vi "Copy Builds To NIVS Dir.vi"(5 "Files Generated by Build":path[](array[path]), 6 "Top Level/Always Included VIs":path[](array[path]), 7 "Destination Path":path, 8 "error in (no error)":errorcluster, 9 "Target Name":string, 10 "Build Specification Name":string, 11 "Project Path":path) -> (0 "error out":errorcluster)   [LabVIEW 2020]
uses:
  <vilib>/Utility/sysdir.llb/System Directory Type.ctl
  <vilib>/regexp/Match Regular Expression.xnode
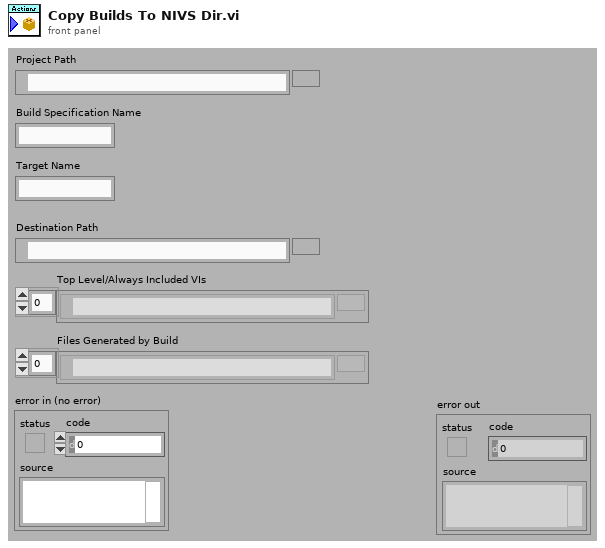
[diagram p1: front panel]
types:
  T1 = typedef "System Directory Type.ctl" = i32
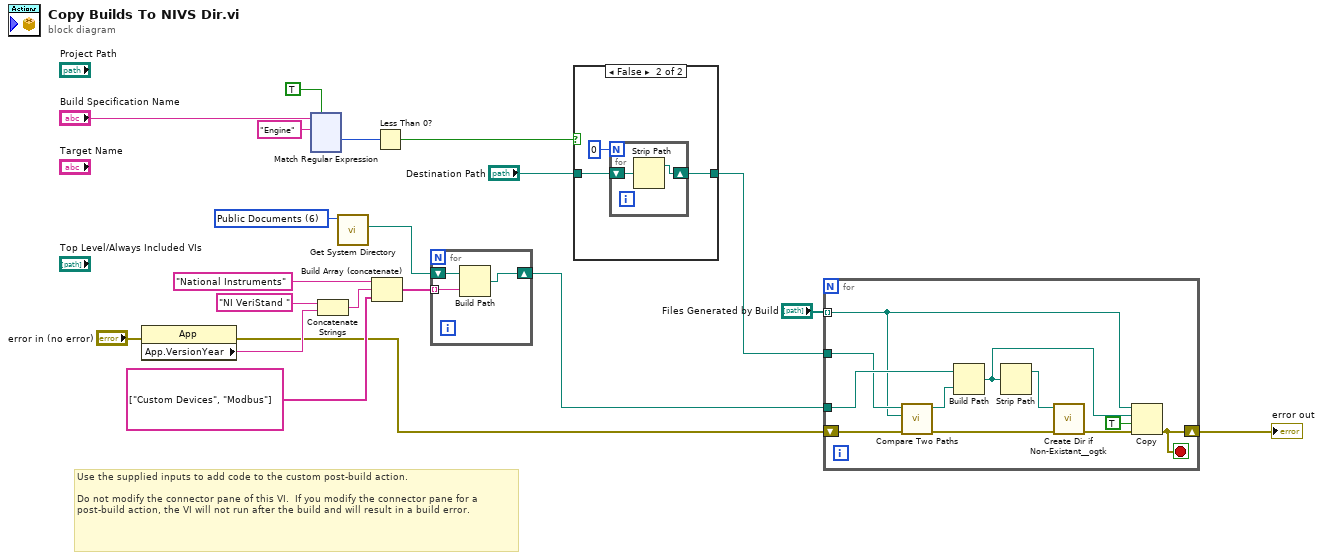
[diagram p0: block diagram]
diagram:
  w19 = T1 6 items=["User Home"=0, "User Desktop"=1, "User Documents"=2, "User Application Data"=3, "User Preferences"=4, "User Temporary"=5, "Public Documents"=6, "Public Application Data"=7, "Public Preferences"=8, "Public Cache"=13, "System Core Libraries"=9, "System Installed Libraries"=10, "Application Files"=11, "Boot Volume Root"=12] ("system directory type")
  # "Use the supplied inputs to add code to the custom post-build action.\n\nDo not modify the connector pane of this VI.  If you modify the connector pane for a post-build action, the VI will not run after the build and will result in a build error."
  n1 = property class="App"(error in="error in (no error)") -> (error out=w7:errorcluster, "App.VersionYear"=w15:string)  [unwired: 1 in, 1 out]
  n2 = xnode "Match Regular Expression"("input string"="Build Specification Name", "regular expression"="Engine", "ignore case? (F)"=TRUE) -> ("offset past match"=w1:i32)  [unwired: 3 in, 4 out]
  n3 = Concatenate Strings("NI VeriStand " ("name or relative path"), w15) -> (w13:string)
  n4 = call <vilib>:"Get System Directory.vi"("system directory type"=w19) -> ("system directory"=w18:path)  [unwired: 10 in]
  n5 = Build Array (concatenate)("National Instruments" ("name or relative path"), w13, string[] ["Custom Devices", "Modbus"]) -> (w11:string[])
  n6 = Less Than 0?(x=w1) -> (x < 0?=w2:bool)
  n7 = for {
    shift-right: [w22] -> w6
    shift-left: w18 -> [w23]
    tunnel: w11 -> [w21] mode=indexing
    n8 = Build Path(base path=w23, name or relative path=w21) -> (appended path=w22:path)
  }
  n9 = case shown="False" w2 {
    tunnel: [w24 w25] -> w9
    tunnel: "Destination Path" -> [w24 w27]
    frame True {
    }
    frame False {
      n10 = for {
        N: 0 -> [_]
        shift-right: [w28] -> w25
        shift-left: w27 -> [w29]
        n11 = Strip Path(path=w29) -> (stripped path=w28:path)  [unwired: 1 out]
      }
    }
  }
  n12 = for {
    shift-right: [w35] -> w10
    shift-left: w7 -> [w39]
    tunnel: "Files Generated by Build" -> [w34] mode=indexing
    tunnel: w6 -> [w38]
    tunnel: w9 -> [w36]
    stop <- w35 stop-if-true
    n13 = call <vilib>:"Compare Two Paths.vi"("error in (no error)"=w39, "Path 2"=w34, "Path 1"=w36) -> ("error out"=w33:errorcluster, "Relative Path from 1 to 2"=w37:path)  [unwired: 5 in, 2 out]
    n14 = Build Path(base path=w38, name or relative path=w37) -> (appended path=w30:path)
    n15 = Strip Path(path=w30) -> (stripped path=w32:path)  [unwired: 1 out]
    n16 = call <userlib>:"Create Dir if Non-Existant__ogtk.vi"("error in (no error)"=w33, "Directory Path"=w32) -> ("error out"=w31:errorcluster)  [unwired: 7 in, 2 out]
    n17 = Copy(8:w31, 9:TRUE ("overwrite (F)"), 10:w30, 11:w34) -> (0:w35:errorcluster)  [unwired: 1 in, 2 out]
  }
  "error out" <- w10
